vi "LabvolutionSubmoduleCheck_Item_OnCommand.vi"(10 "Command ID":string, 11 "Object":T1) -> ()   [LabVIEW 2018]
uses:
  <resource>/Framework/Providers/API/ItemRef.ctl
panel:
  out "error out":errorcluster
  in  "error in":errorcluster
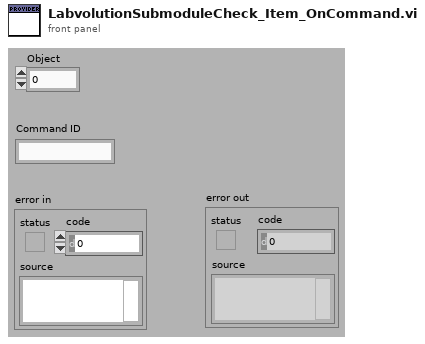
[diagram p1: front panel]
types:
  T1 = typedef "ItemRef.ctl" = u64
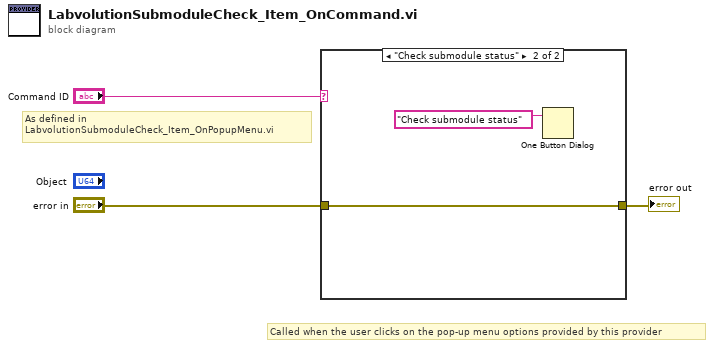
[diagram p0: block diagram]
diagram:
  # "As defined in \nLabvolutionSubmoduleCheck_Item_OnPopupMenu.vi"
  # "Called when the user clicks on the pop-up menu options provided by this provider"
  n1 = case shown="\"Check submodule status\"" "Command ID" {
    tunnel: "error in" -> [w4 w5]
    tunnel: [w4 w5] -> w1
    frame Default {
    }
    frame "Check submodule status" {
      n2 = One Button Dialog(message="Check submodule status") -> ()  [unwired: 1 in, 1 out]
    }
  }
  "error out" <- w1
